vi "RTUserInterface.vi"(8 "error in (no error)":errorcluster) -> (0 "error out":errorcluster)   [LabVIEW 2016]
uses:
  controls/SwitchStates.ctl
  controls/MotorSetStates.ctl
  controls/RT-Variables.lvlib
panel:
  in  "EnvCoverPos":T1 caption="Position"
  out "CalInject out":bool caption="Status"
  out "EnvCover":bool caption="Status"
  out "RemoteState":T2
  in  "stop":bool
  # "Env. Cover"
  # "Cal. Inject"
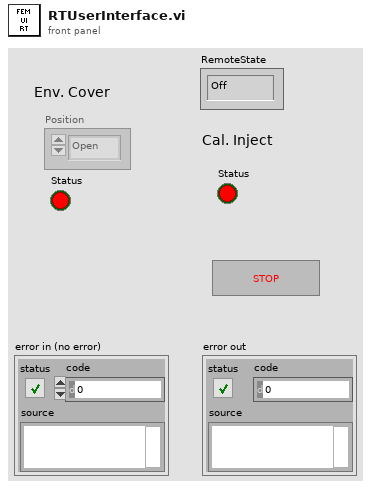
[diagram p1: front panel]
types:
  T1 = typedef "RT-Variables.lvlib/MotorSetStates.ctl" = enum16{"Open", "Close"}
  T2 = typedef "RT-Variables.lvlib/SwitchStates.ctl" = enum16{"Off", "Local", "Remote"}
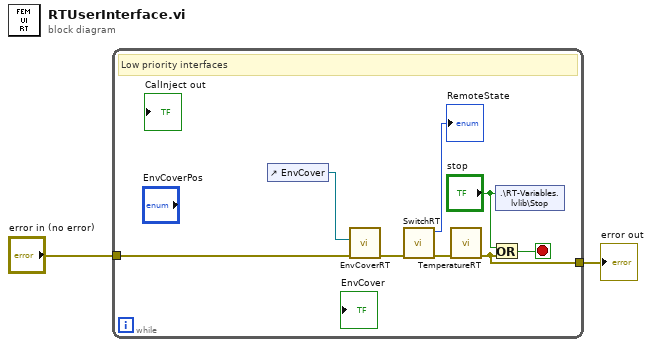
[diagram p0: block diagram]
diagram:
  n1 = while {
    tunnel: "error in (no error)" -> [w3]
    tunnel: [w7] -> w1
    stop <- w10 stop-if-true
    # "Low priority interfaces"
    n2 = control-ref of="EnvCover"() -> (w6:refnum<vi>)
    n3 = call "EnvCoverRT.vi"("error in (no error)"=w3, "Boolean in"=w6) -> ("error out"=w5:errorcluster)  [unwired: 8 in]
    n4 = call "SwitchRT.vi"("error in (no error)"=w5) -> ("error out"=w9:errorcluster, "RemoteState"=→"RemoteState":T2)  [unwired: 9 in]
    n5 = call "TemperatureRT.vi"("error in (no error)"=w9) -> ("error out"=w7:errorcluster)  [unwired: 10 in]
    n6 = Or(x="stop", y=w7) -> (x .or. y?=w10:bool)
    n7 = shared-variable ".\\RT-Variables.lvlib\\Stop"("stop") -> ()  [unwired: 1 in, 1 out]
  }
  "error out" <- w1
